vi "Get Restarts Data.vi"(10 "error in":errorcluster, 11 "Path":path) -> (0 "Cogging Data":cluster{"CogEvents":i32[], "CogLimits":i32[]}, 1 "Restarts Limits":T3={"High Limits:"=[30, 30, 30, 30, 30, 30], "Low Limits:"=[30, 30, 30, 30, 30, 30]}, 2 "Actual Starts":T1, 3 "Restarts Cluster":T2, 4 "error out":errorcluster)   [LabVIEW 2013]
uses:
  Type Defs/Restarts Limits.ctl
  Type Defs/Restarts Cluster.ctl
  Type Defs/Actual Starts.ctl
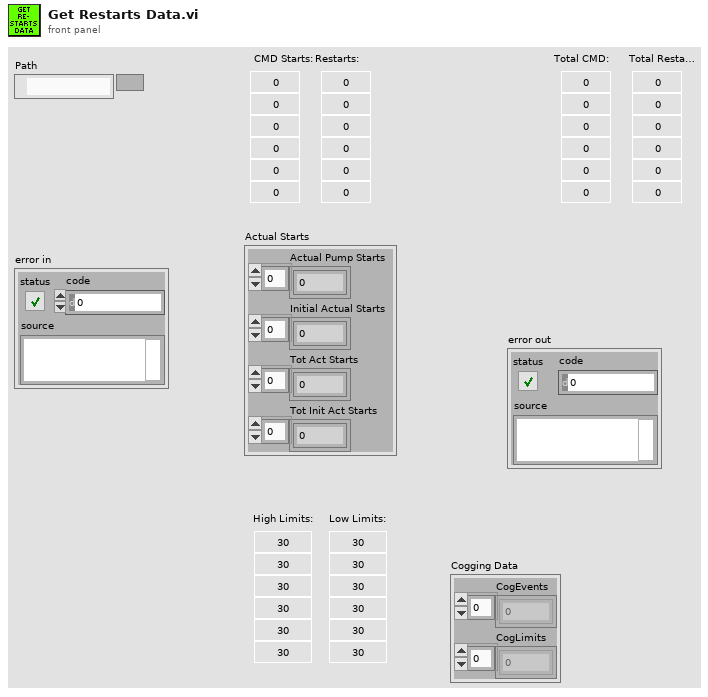
[diagram p1: front panel]
types:
  T1 = typedef "Actual Starts.ctl" = cluster{"Actual Pump Starts":i32[], "Initial Actual Starts":i32[], "Tot Act Starts":i32[], "Tot Init Act Starts":i32[]}
  T2 = typedef "Restarts Cluster.ctl" = cluster{"CMD Starts:":i32[], "Restarts:":i32[], "Total CMD:":i32[], "Total Restarts:":i32[]}
  T3 = typedef "Restarts Limits.ctl" = cluster{"High Limits:":i32[], "Low Limits:":i32[]}
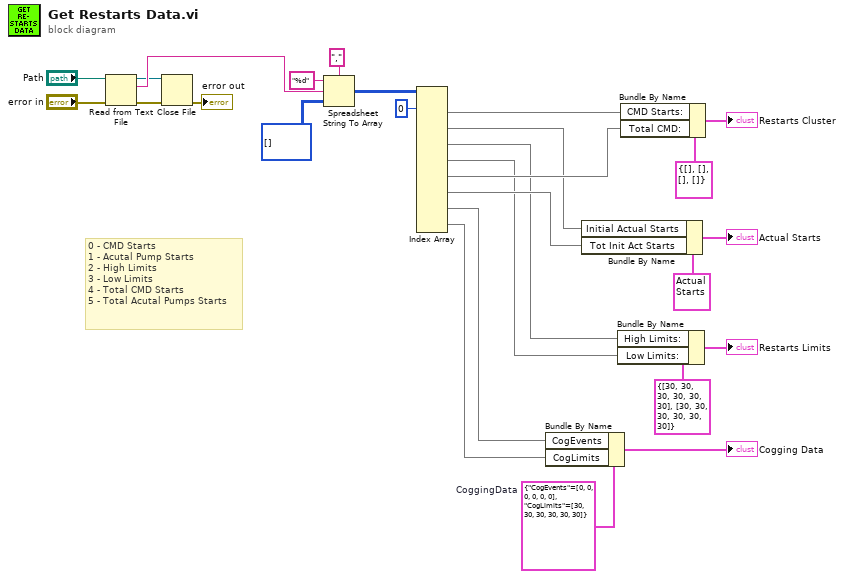
[diagram p0: block diagram]
diagram:
  w6 = cluster{"CogEvents":i32[], "CogLimits":i32[]} {"CogEvents"=[0, 0, 0, 0, 0, 0], "CogLimits"=[30, 30, 30, 30, 30, 30]}  # CoggingData
  # "0 - CMD Starts\n1 - Acutal Pump Starts\n2 - High Limits\n3 - Low Limits\n4 - Total CMD Starts\n5 - Total Acutal Pumps Starts"
  n1 = Read from Text File(file (use dialog)="Path", error in="error in") -> (refnum out=w24:refnum<file>, text=w25:string, error out=w23:errorcluster)  [unwired: 2 in, 1 out]
  n2 = Close File(refnum=w24, error in=w23) -> (error out=→"error out":errorcluster)  [unwired: 1 out]
  n3 = Spreadsheet String To Array(delimiter (Tab)=",", format string="%d", spreadsheet string=w25, array type (2D Dbl)=i32[][] []) -> (array=w20:i32[][])
  n4 = Index Array(array=w20, index (row) #1=0 ("index (row)")) -> (element #1=w17:i32[], element #2=w12:i32[], element #3=w9:i32[], element #4=w8:i32[], element #5=w15:i32[], element #6=w11:i32[], element #7=w5:i32[], element #8=w4:i32[])  [unwired: 15 in]
  n5 = Bundle By Name(cluster=w6, "CogEvents"=w5, "CogLimits"=w4) -> (→"Cogging Data":cluster{"CogEvents":i32[], "CogLimits":i32[]})
  n6 = Bundle By Name(cluster=T1 {"Actual Pump Starts"=[0, 0, 0, 0, 0, 0], "Initial Actual Starts"=[0, 0, 0, 0, 0, 0], "Tot Act Starts"=[0, 0, 0, 0, 0, 0], "Tot Init Act Starts"=[0, 0, 0, 0, 0, 0]} ("Actual Starts"), "Initial Actual Starts"=w12, "Tot Init Act Starts"=w11) -> (→"Actual Starts":T1)
  n7 = Bundle By Name(cluster=T3 {"High Limits:"=[30, 30, 30, 30, 30, 30], "Low Limits:"=[30, 30, 30, 30, 30, 30]} ("Restarts Limits"), "High Limits:"=w9, "Low Limits:"=w8) -> (→"Restarts Limits":T3)
  n8 = Bundle By Name(cluster=T2 {"CMD Starts:"=[], "Restarts:"=[], "Total CMD:"=[], "Total Restarts:"=[]} ("Restarts Cluster"), "CMD Starts:"=w17, "Total CMD:"=w15) -> (→"Restarts Cluster":T2)
